vi "SUM_BLANK_CHANNELS.vi"(8 "error in":errorcluster, 11 "connection ID in":refnum<k5>) -> (0 "error out":errorcluster, 3 "connection ID out":refnum<k5>)   [LabVIEW 2012]
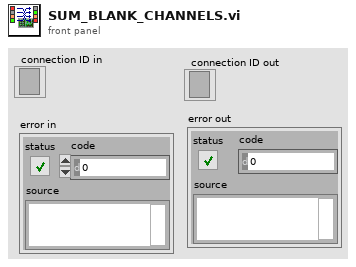
[diagram p1: front panel]
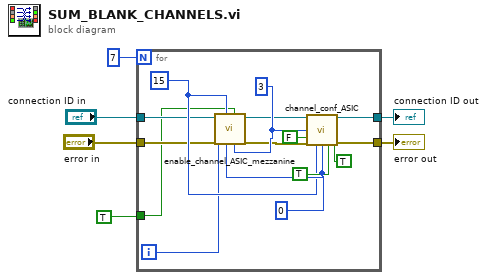
[diagram p0: block diagram]
diagram:
  n1 = for {
    N: 7 -> [_]
    tunnel: "connection ID in" -> [w11]
    tunnel: "error in" -> [w12]
    tunnel: [w10] -> w2
    tunnel: [w9] -> w1
    tunnel: TRUE ("Sum/Maj") -> [w8]
    i -> [w7]
    w18 = u32 0 ("Ib_ClipVb")
    w17 = u32 3 ("Clip_sel_b")
    w16 = u32 15 ("Att gain")
    n2 = call "enable_channel_ASIC_mezzanine.vi"("Clip_sel_b"=w17, "maj/sum"=w8, "Ib_clipVb"=w18, "Att gain"=w16, "error in"=w12, "Channel"=w7, "connection ID"=w11) -> ("error out"=w13:errorcluster, "connection ID out"=w14:refnum<k5>)  [unwired: 2 in, 1 out]
    n3 = call "channel_conf_ASIC.vi"("connection ID"=w14, "Clip_sel_b"=w17, "CompBuf_en_b"=FALSE, "error out"=w13, "Att gain"=w16, "Ib_ClipVb"=w18, "Clip_en_b"=TRUE, "Att_en_b"=TRUE) -> ("connection ID out"=w9:refnum<k5>, "error out 2"=w10:errorcluster)  [unwired: 3 in, 3 out]
  }
  "error out" <- w2
  "connection ID out" <- w1
